vi "Measurement.Init.vi"(8 "error in (no error)":errorcluster, 10 "timeout (5000 ms)":i32=5000, 11 "Measurement.Free in":refnum<class "Measurement.Free.lvclass">) -> (0 "error out":errorcluster, 2 "Result":bool, 3 "Measurement.Free out":refnum<class "Measurement.Free.lvclass">)   [LabVIEW 2017, in "Measurement.Free.lvclass"]
uses:
  Measurement.Free.lvclass
  OPA/OPA.lvclass
  D:/upwork/Laser Measurement Tool/Laser/project/Subsystems/Device/Device.lvclass
  OPM/OPM.lvclass
  LIA/LIA.lvclass
  SMU/SMU.lvclass
  Device/Device.lvclass
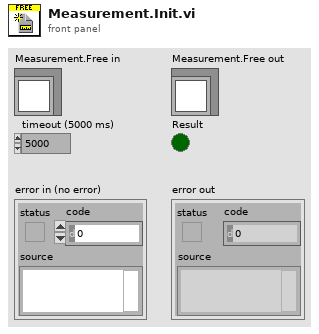
[diagram p1: front panel]
types:
  T1 = typedef "Measurement.Free.lvclass/Configuration--Cluster.ctl" = cluster{"Measurement.Type":enum16{"Free", "I/V Curve", "Wavelength sweeping", "Photocurrent mapping"}, "Hardware":T2}
  T2 = typedef "Measurement.Free.lvclass/Configuration.Hardware--Cluster.ctl" = cluster{"SMU":T3, "LIA":T5, "OPM":T7, "OPA":T9}
  T3 = typedef "Measurement.lvclass/Configuration.SMU--Cluster.ctl" = cluster{"Enable":bool, "SMU Model":string, "Configuration":T4}
  T4 = typedef "SMU.lvclass/Configuration--Cluster.ctl" = cluster{"VISA Resource":string, "Channel":string}
  T5 = typedef "Measurement.lvclass/Configuration.LIA--Cluster.ctl" = cluster{"Enable":bool, "LIA Model":string, "Configuration":T6}
  T6 = typedef "LIA.lvclass/Configuration--Cluster.ctl" = cluster{"VISA Resource":string}
  T7 = typedef "Measurement.lvclass/Configuration.OPM--Cluster.ctl" = cluster{"Enable":bool, "OPM Model":string, "Configuration":T8}
  T8 = typedef "OPM.lvclass/Configuration--Cluster.ctl" = cluster{"VISA Resource":string}
  T9 = typedef "Measurement.lvclass/Configuration.OPA--Cluster.ctl" = cluster{"Enable":bool, "OPA Model":string, "Configuration":T10}
  T10 = typedef "OPA.lvclass/Configuration--Cluster.ctl" = cluster{"Serial Number":string}
  T11 = typedef "Measurement.Free.lvclass/Dependencies--Cluster.ctl" = cluster{"SMU":refnum<class "SMU.lvclass">, "LIA":refnum<class "LIA.lvclass">, "OPM":refnum<class "OPM.lvclass">, "OPA":refnum<class "OPA.lvclass">}
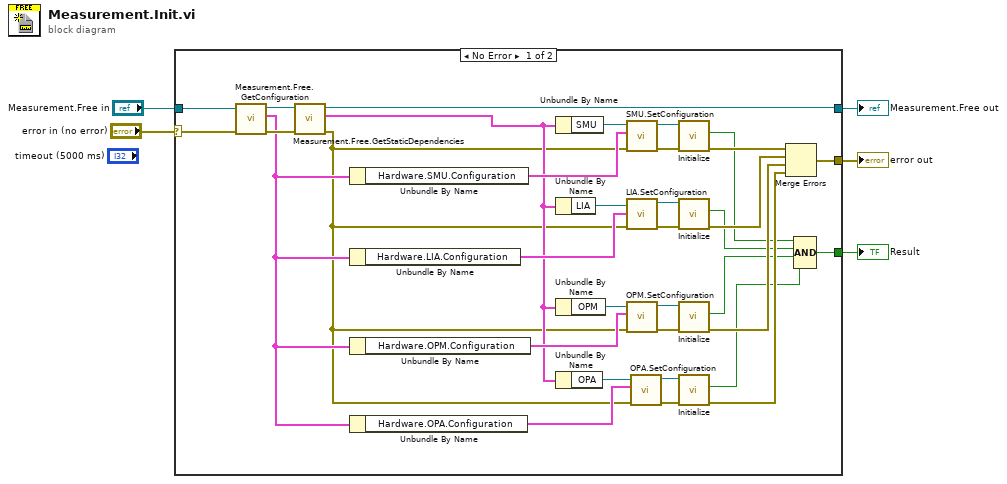
[diagram p0: block diagram]
diagram:
  n1 = case shown="No Error" "error in (no error)" {
    selector: "error in (no error)" -> [w37 w41]
    tunnel: [w29 w41] -> w1
    tunnel: [w31 w40] -> w3
    tunnel: "Measurement.Free in" -> [w39 w40]
    tunnel: [w6 _] -> w2
    frame No Error {
      n2 = call "Measurement.Free.GetConfiguration.vi"("error in (no error)"=w37, "Measurement.Free"=w39) -> ("error out"=w36:errorcluster, "Configuration"=w18:T1, "Measurement.Free out"=w38:refnum<class "Measurement.Free.lvclass">)  [unwired: 7 in]
      n3 = call "Measurement.Free.GetStaticDependencies.vi"("error in (no error)"=w36, "Measurement.Free"=w38) -> ("error out"=w14:errorcluster, "Dependencies"=w17:T11, "Measurement.Free out"=w31:refnum<class "Measurement.Free.lvclass">)  [unwired: 7 in]
      n4 = Unbundle By Name(w18) -> ("Hardware.SMU.Configuration"=w34:T4)
      n5 = Unbundle By Name(w18) -> ("Hardware.LIA.Configuration"=w27:T6)
      n6 = Unbundle By Name(w18) -> ("Hardware.OPM.Configuration"=w22:T8)
      n7 = Unbundle By Name(w18) -> ("Hardware.OPA.Configuration"=w15:T10)
      n8 = Unbundle By Name(w17) -> ("SMU"=w35:refnum<class "SMU.lvclass">)
      n9 = Unbundle By Name(w17) -> ("LIA"=w28:refnum<class "LIA.lvclass">)
      n10 = Unbundle By Name(w17) -> ("OPM"=w23:refnum<class "OPM.lvclass">)
      n11 = Unbundle By Name(w17) -> ("OPA"=w16:refnum<class "OPA.lvclass">)
      n12 = call "SMU.SetConfiguration.vi"("error in (no error)"=w14, "Configuration"=w34, "SMU"=w35) -> ("error out"=w32:errorcluster, "SMU out"=w33:refnum<class "SMU.lvclass">)  [unwired: 7 in]
      n13 = call "LIA.SetConfiguration.vi"("error in (no error)"=w14, "Configuration"=w27, "LIA"=w28) -> ("error out"=w26:errorcluster, "LIA out"=w25:refnum<class "LIA.lvclass">)  [unwired: 7 in]
      n14 = call "OPM.SetConfiguration.vi"("error in (no error)"=w14, "Configuration"=w22, "PM"=w23) -> ("error out"=w20:errorcluster, "PM out"=w21:refnum<class "OPM.lvclass">)  [unwired: 7 in]
      n15 = call "OPA.SetConfiguration.vi"("error in (no error)"=w14, "Configuration"=w15, "OPA"=w16) -> ("error out"=w13:errorcluster, "OPA out"=w12:refnum<class "OPA.lvclass">)  [unwired: 7 in]
      n16 = call "Initialize.vi"("error in (no error)"=w32, "Device in"=w33) -> ("error out"=w30:errorcluster, "Result"=w10:bool)  [unwired: 7 in, 1 out]
      n17 = call "Initialize.vi"("error in (no error)"=w26, "Device in"=w25) -> ("error out"=w24:errorcluster, "Result"=w9:bool)  [unwired: 7 in, 1 out]
      n18 = call "Initialize.vi"("error in (no error)"=w20, "Device in"=w21) -> ("error out"=w19:errorcluster, "Result"=w8:bool)  [unwired: 7 in, 1 out]
      n19 = call "Initialize.vi"("error in (no error)"=w13, "Device in"=w12) -> ("error out"=w11:errorcluster, "Result"=w7:bool)  [unwired: 7 in, 1 out]
      n20 = Merge Errors(w30, w24, w19, w11) -> (w29:errorcluster)
      n21 = Compound Arithmetic op=AND(w10, w9, w8, w7) -> (w6:bool)
    }
    frame Error {
    }
  }
  "error out" <- w1
  "Measurement.Free out" <- w3
  "Result" <- w2
